vi "read_attributes.vi"(8 "error in (no error)":errorcluster, 11 "GradientBoostingClassifier in":refnum<class "GradientBoostingClassifier.lvclass">) -> (0 "error out":errorcluster, 2 "attributes":T1, 3 "GradientBoostingClassifier out":refnum<class "GradientBoostingClassifier.lvclass">)   [LabVIEW 2020, in "GradientBoostingClassifier.lvclass"]
uses:
  GradientBoostingClassifier.lvclass
  Controls/gradient_boosting_classifier_attributes.ctl
  GradientBoostingClassifier.lvclass/GradientBoostingClassifier.ctl
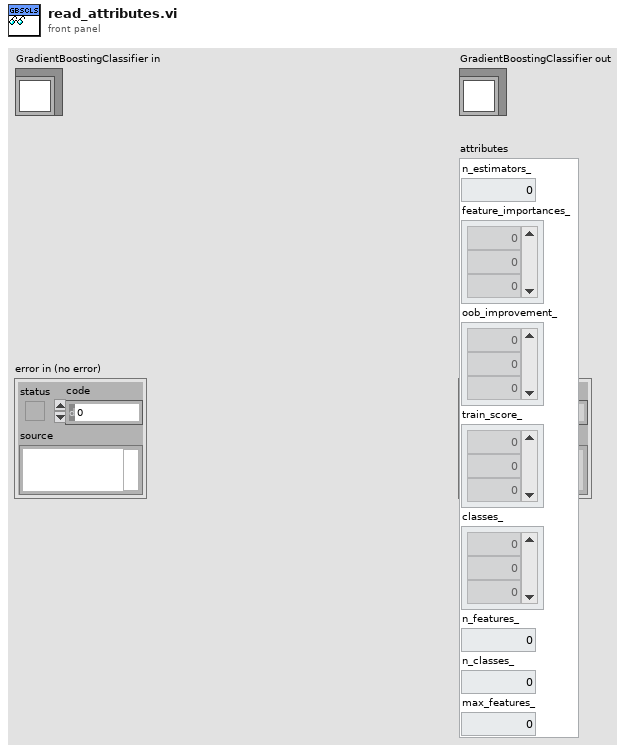
[diagram p1: front panel]
types:
  T1 = typedef "gradient_boosting_classifier_attributes.ctl" = cluster{"n_estimators_":dbl, "feature_importances_":dbl[], "oob_improvement_":dbl[], "train_score_":dbl[], "classes_":dbl[], "n_features_":dbl, "n_classes_":dbl, "max_features_":dbl}
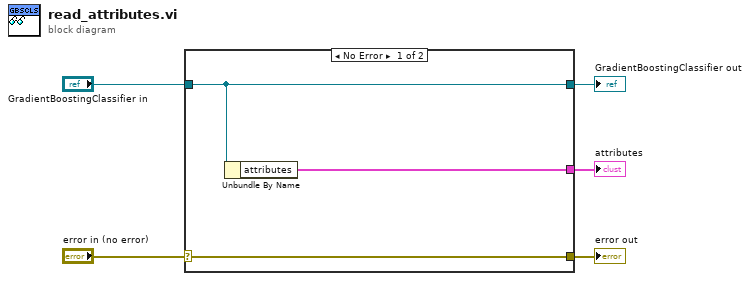
[diagram p0: block diagram]
diagram:
  n1 = case shown="No Error" "error in (no error)" {
    selector: "error in (no error)" -> [w8 w9]
    tunnel: [w8 w9] -> w4
    tunnel: [w7 w10] -> w2
    tunnel: "GradientBoostingClassifier in" -> [w7 w10]
    tunnel: [w6 _] -> w1
    frame No Error {
      n2 = Unbundle By Name(w7) -> ("attributes"=w6:T1)
    }
    frame Error {
    }
  }
  "error out" <- w4
  "GradientBoostingClassifier out" <- w2
  "attributes" <- w1
